vi "GetMACFromDB.vi"(8 "error in":errorcluster, 9 "all string":string, 10 "Procedure name":string, 11 "DSN name":string) -> (0 "error out":errorcluster caption="错误输出", 2 "MAC":string[](array[string]))   [LabVIEW 2013]
uses:
  <vilib>/addons/database/Connection.llb/DB Tools Open Connec (String).vi
  <vilib>/addons/database/Connection.llb/Conn Execute.vi
  <vilib>/addons/database/Recordset.llb/Rec Fetch Recordset Data (R).vi
  <vilib>/addons/database/Recordset.llb/Rec Destroy - Connection.vi
  <vilib>/addons/database/NI_Database_API.lvlib
panel:
  out "连接的字符串":string
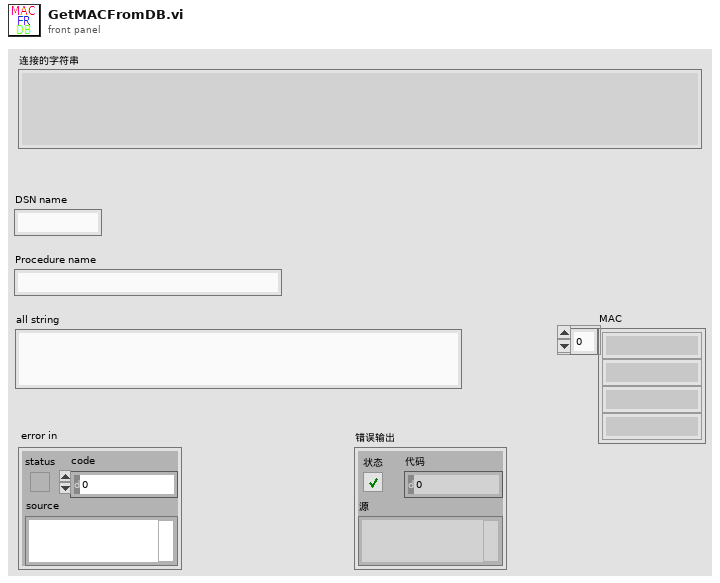
[diagram p1: front panel]
types:
  T1 = typedef "NI_Database_API.lvlib/Conn ObjectReference.ctl" = refnum<k1>
  T2 = typedef "NI_Database_API.lvlib/Rec ObjectReference.ctl" = refnum<k1>
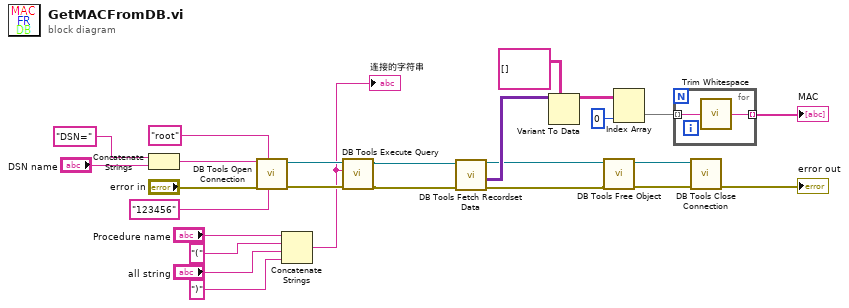
[diagram p0: block diagram]
diagram:
  n1 = Concatenate Strings("DSN=", "DSN name") -> (w16:string)
  n2 = call-poly <vilib>:"DB Tools Open Connection.vi"("password"="123456" ("userID"), "userID"="root", "error in (no error)"="error in", "connection information"=w16) -> ("error out"=w26:errorcluster, "connection reference"=w25:T1)  [unwired: 4 in]
  n3 = Concatenate Strings("Procedure name", "(", "all string", ")") -> (w21:string)
  "连接的字符串" <- w21
  n4 = call-poly <vilib>:"DB Tools Execute Query.vi"("error in (no error)"=w26, "SQL query"=w21, "connection reference"=w25) -> ("error out"=w9:errorcluster, "recordset reference"=w10:T2)  [unwired: 5 in]
  n5 = call-poly <vilib>:"DB Tools Fetch Recordset Data.vi"("error in (no error)"=w9, "recordset reference"=w10) -> ("error out"=w7:errorcluster, "recordset data"=w12:variant[][], "recordset reference out"=w8:T2)  [unwired: 3 in]
  n6 = Variant To Data(type=string[][] [], Variant=w12) -> (data=w6:string[][])  [unwired: 1 in, 1 out]
  n7 = call-poly <vilib>:"DB Tools Free Object.vi"("error in (no error)"=w7, "recordset reference"=w8) -> ("error out"=w23:errorcluster, "connection reference"=w24:T1)  [unwired: 8 in]
  n8 = Index Array(array=w6, index (col)=0 ("索引 (行)")) -> (element=w2:string[])  [unwired: 1 in]
  n9 = for {
    tunnel: w2 -> [w28] mode=indexing
    tunnel: [w27] -> w1 mode=indexing
    n10 = call <vilib>:"Trim Whitespace.vi"("string"=w28) -> ("trimmed string"=w27:string)  [unwired: 1 in]
  }
  "MAC" <- w1
  n11 = call <vilib>:"DB Tools Close Connection.vi"("error in (no error)"=w23, "connection reference"=w24) -> ("error out"=→"error out":errorcluster)  [unwired: 5 in]
